vi "RegisterEngine.vi"(8 "error in (no error)":errorcluster, 11 "IAmEngine":refnum<class "IAmEngine.lvclass">) -> (0 "error out":errorcluster)   [LabVIEW 2024, in "GLF.lvlib" / "DVRHandler.lvlib"]
uses:
  DVRHandler.lvlib
  IAmEngine/IAmEngine.lvclass
  Action--enum.ctl
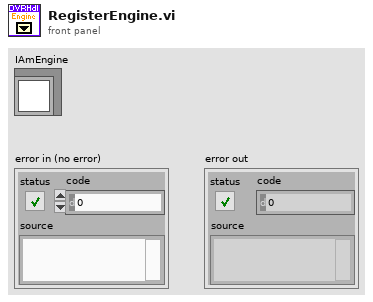
[diagram p1: front panel]
types:
  T1 = typedef "GLF.lvlib/DVRHandler.lvlib/Action--enum.ctl" = enum16{"Set IAmEngine"}
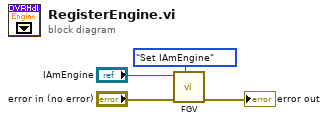
[diagram p0: block diagram]
diagram:
  n1 = call "FGV.vi"("Action"=Action--enum."Set IAmEngine", "error in (no error)"="error in (no error)", "IAmEngine"="IAmEngine") -> ("error out"=→"error out":errorcluster)  [unwired: 8 in]
